vi "LeakageVSTemp-Time_Keithley6517A.vi"() -> ()   [LabVIEW 2010]
uses:
  <vilib>/Instr/_visa.llb/VISA Configure Serial Port (Instr).vi
  <vilib>/Utility/file.llb/Write To Spreadsheet File (DBL).vi
  Instance          14 32Saved   K vs Temp - freq (4284A) .vi
  Instance          10 32Saved   K vs Temp - freq (4284A) .vi
  Instance          25 32Saved   K vs Temp - freq (4284A) .vi
  Instance          24 32Saved   K vs Temp - freq (4284A) .vi
  Instance          26 32Saved   K vs Temp - freq (4284A) .vi
panel:
  in  "Time":dbl[](array[numeric])
  out "?":string="Current"
  in  "control":sgl[](array[numeric]) format="%.2f"
  out "Test Data":sgl[][](array[numeric])=[[1.0, 2.2355776e-13]] format="%.6p"
  out "error out":T1
  in  "error in":T1
  in  "Interval(secs)":sgl=1.0 min=0 max=9999.9 step=0.1 format="%.1f"
  in  "Number of Points":sgl=1.0 min=0 max=9999.9 step=0.1 format="%.1f"
  in  "Bias Voltage":sgl=1.0 min=-1000 max=1000 step=0.1 format="%.1f"
  in  "Current (nA)":dbl[](array[numeric])
  in  "Current (nA)":dbl[](array[numeric])
  in  "Temperature":dbl[](array[numeric])
  in  "Start":bool
  out "Thickness":dbl
  out "Area":dbl
  in  "stop":bool
  out "Temp25Hz":dbl format="%#_3g"
  out "Current (nA) vs. Time":cluster{"Y":dbl[], "Y":dbl[]}[](graph)
  out "Current (nA) vs. Temperature":cluster{"Y":dbl[], "Y":dbl[]}[](graph)
  in  "Comment (Sample's Name, compositions, whatever you want,..)":string
  in  "Thickness (mm)":dbl
  in  "Diameter (mm)":dbl
  in  "Path & File Name (*.txt)":path
  # "Temperature (C)"
  # "Sample Details"
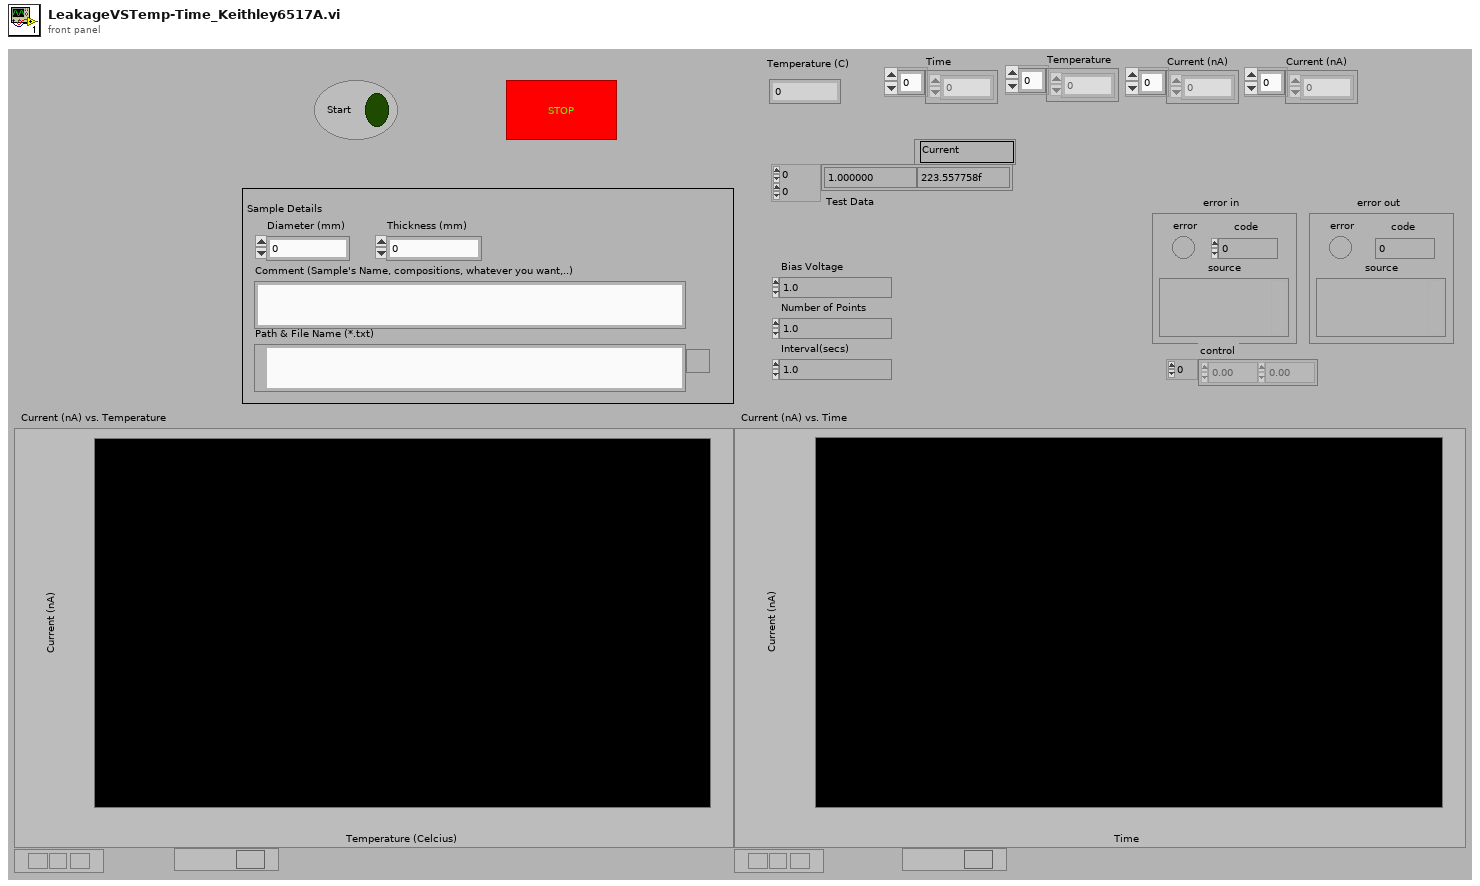
[diagram p1: front panel]
types:
  T1 = cluster{"error":bool, "code":i32, "source":string}
  T2 = cluster{"second":i32, "minute":i32, "hour":i32, "day of month":i32, "month":i32, "year":i32, "day of week":i32, "day of year":i32, "is DST":i32}
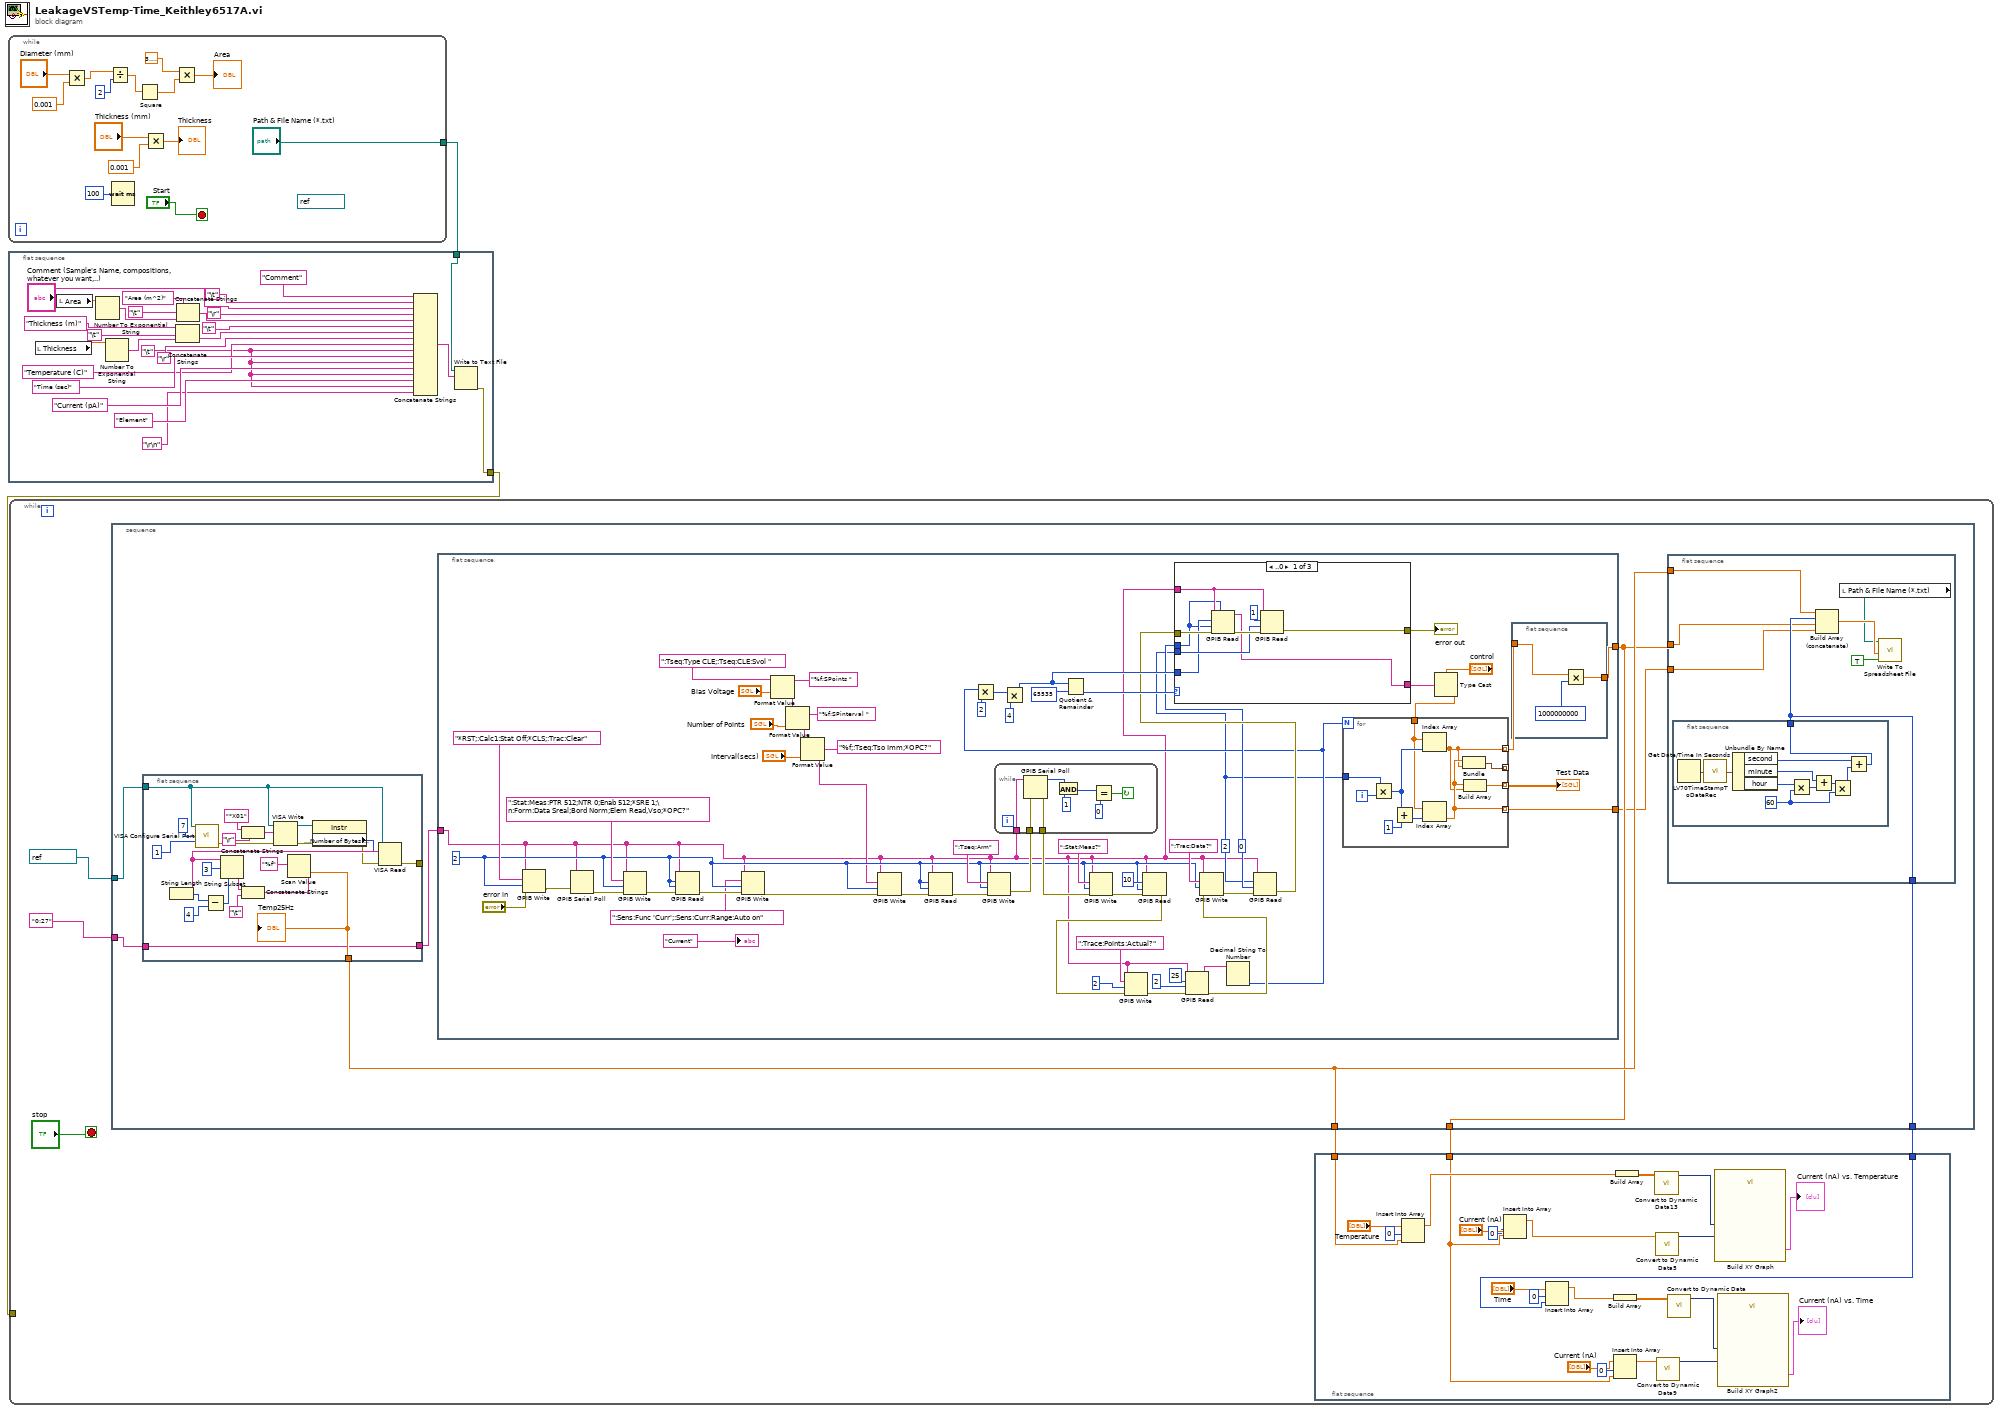
[diagram p0: block diagram]
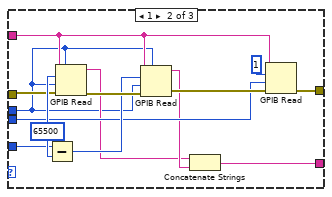
[diagram p2: hidden frame]
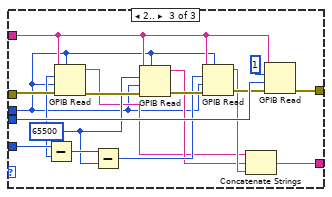
[diagram p3: hidden frame]
diagram:
  n1 = while {
    tunnel: ["Path & File Name (*.txt)"] -> w2
    stop <- "Start" stop-if-true
    (unwired) refnum<visa-resource-name> "COM1" ("VISA Omega (Serial - COM1)")
    n2 = Multiply(x="Diameter (mm)", y=0.001) -> (x*y=w11:dbl)
    n3 = Divide(x=w11, y=2) -> (x/y=w6:dbl)
    n4 = Wait (ms)(milliseconds to wait=u32 100) -> ()  [unwired: 1 out]
    n5 = Square(x=w6) -> (x^2=w7:dbl)
    n6 = Multiply(x="Thickness (mm)", y=0.001) -> (x*y=→"Thickness":dbl)
    n7 = Multiply(x=3.141592653589793, y=w7) -> (x*y=→"Area":dbl)
  }
  n8 = flat-sequence {
    tunnel: w2 -> [w36]
    tunnel: [w34] -> w1
    frame #0 {
      w18 = "\t"
      n9 = local read "Thickness"() -> (w40:dbl)
      n10 = local read "Area"() -> (w41:dbl)
      n11 = Number To Exponential String(number=w41) -> (E-format string=w33:string)  [unwired: 3 in]
      n12 = Number To Exponential String(number=w40) -> (E-format string=w31:string)  [unwired: 3 in]
      n13 = Concatenate Strings("Thickness (m)" ("string"), "\t", w31) -> (w29:string)
      n14 = Concatenate Strings("Area (m^2)" ("string"), "\t", w33) -> (w37:string)
      n15 = Concatenate Strings("Comment" ("string"), "\t", "Comment (Sample's Name, compositions, whatever you want,..)", "\r", w37, "\t", w29, "\r", "Temperature (C)" ("string"), w18, "Time (sec)" ("string"), w18, "Current (pA)" ("string"), w18, "Element" ("string"), w18, "\r\n") -> (w35:string)
      n16 = Write to Text File(file (use dialog)=w36, text=w35) -> (error out=w34:errorcluster)  [unwired: 2 in, 2 out]
    }
  }
  n17 = while {
    tunnel: w1 -> [_]
    stop <- "stop" stop-if-true
    n18 = stacked-sequence {
      tunnel: refnum<visa-resource-name> "COM1" ("VISA Omega (Serial - COM1)") -> [w77]
      tunnel: "0:27" -> [w76]
      tunnel: [w74] -> w44
      tunnel: [w73] -> w43
      tunnel: [w71] -> w42
      frame #0 {
        n19 = flat-sequence {
          tunnel: w77 -> [w217]
          tunnel: [w216] -> _
          tunnel: [w215] -> w74
          tunnel: w76 -> [w214]
          tunnel: [w214] -> w75
          frame #0 {
            n20 = call-poly "VISA Configure Serial Port"("VISA resource name"=w217, "data bits (8)"=7, "parity (0:none)"=1) -> ("error out"=w222:errorcluster)  [unwired: 11 in, 1 out]
            n21 = Concatenate Strings("*X01", "\r") -> (w225:string)
            n22 = VISA Write(VISA resource name=w217, write buffer=w225, error in (no error)=w222) -> (VISA resource name out=w236:refnum<visa-resource-name>, error out=w226:errorcluster)  [unwired: 1 out]
            n23 = property class="Instr"(reference=w236, error in=w226) -> (error out=w227:errorcluster, "Serial Settings:Number of Bytes at Serial Port"=w228:u32)  [unwired: 1 out]
            n24 = VISA Read(VISA resource name=w217, byte count=w228, error in (no error)=w227) -> (read buffer=w229:string, error out=w216:errorcluster)  [unwired: 2 out]
            n25 = String Length(string=w229) -> (length=w231:i32)
            n26 = Subtract(x=w231, y=4) -> (x-y=w233:i32)
            n27 = String Subset(string=w229, offset (0)=3, length (rest)=w233) -> (substring=w234:string)
            n28 = Concatenate Strings(w234, "\t") -> (w218:string)
            n29 = Scan Value(string=w218, format string="%f") -> (value=w215:dbl)  [unwired: 1 in, 1 out]
            "Temp25Hz" <- w215
          }
        }
        n30 = flat-sequence {
          tunnel: w75 -> [w98]
          tunnel: [w97] -> w72
          tunnel: [w95] -> w73
          frame #0 {
            w124 = 0
            w109 = 2
            w102 = 2
            n31 = GPIB Write(0:w98, 1:"*RST;:Calc1:Stat Off;*CLS;:Trac:Clear", 2:w102, 3:"error in") -> (6:w150:errorcluster)  [unwired: 1 in, 1 out]
            n32 = GPIB Serial Poll(0:w98, 1:w150) -> (4:w149:errorcluster)  [unwired: 2 out]
            n33 = GPIB Write(0:w98, 1:":Stat:Meas:PTR 512;NTR 0;Enab 512;*SRE 1;\n:Form:Data Sreal;Bord Norm;Elem Read,Vso;*OPC?", 2:w102, 3:w149) -> (6:w147:errorcluster)  [unwired: 1 in, 1 out]
            n34 = GPIB Read(0:w98, 1:w102, 2:w102, 3:w147) -> (7:w103:errorcluster)  [unwired: 1 in, 2 out]
            n35 = GPIB Write(0:w98, 1:":Sens:Func 'Curr';:Sens:Curr:Range:Auto on", 2:w102, 3:w103) -> (6:w104:errorcluster)  [unwired: 1 in, 1 out]
            n36 = Format Value(string ("")=":Tseq:Type CLE;:Tseq:CLE:Svol ", format string="%f;SPoints ", value (0)="Bias Voltage") -> (output string=w144:string)
            n37 = Format Value(string ("")=w144, format string="%f;SPinterval ", value (0)="Number of Points") -> (output string=w142:string)
            n38 = Format Value(string ("")=w142, format string="%f;:Tseq:Tso Imm;*OPC?", value (0)="Interval(secs)") -> (output string=w99:string)
            n39 = GPIB Write(0:w98, 1:w99, 2:w102, 3:w104) -> (6:w140:errorcluster)  [unwired: 1 in, 1 out]
            n40 = GPIB Read(0:w98, 1:w102, 2:w102, 3:w140) -> (7:w139:errorcluster)  [unwired: 1 in, 2 out]
            n41 = GPIB Write(0:w98, 1:":Tseq:Arm", 2:w102, 3:w139) -> (6:w132:errorcluster)  [unwired: 1 in, 1 out]
            n42 = while {
              tunnel: w132 -> [w209]
              tunnel: [w208] -> w131
              tunnel: w98 -> [w207]
              stop <- w212 continue-if-true
              n43 = GPIB Serial Poll(0:w207, 1:w209) -> (2:w211:i16, 4:w208:errorcluster)  [unwired: 1 out]
              n44 = And(x=w211, y=1) -> (x .and. y?=w206:i32)
              n45 = Equal?(x=w206, y=0) -> (x = y?=w212:bool)
            }
            n46 = GPIB Write(0:w98, 1:":Stat:Meas?", 2:w102, 3:w131) -> (6:w136:errorcluster)  [unwired: 1 in, 1 out]
            n47 = GPIB Read(0:w98, 1:10, 2:w102, 3:w136) -> (7:w117:errorcluster)  [unwired: 1 in, 2 out]
            n48 = GPIB Write(0:w98, 1:":Trace:Points:Actual?", 2:2, 3:w117) -> (6:w120:errorcluster)  [unwired: 1 in, 1 out]
            n49 = GPIB Read(0:w98, 1:25, 2:2, 3:w120) -> (5:w115:string, 7:w116:errorcluster)  [unwired: 1 in, 1 out]
            n50 = GPIB Write(0:w98, 1:":Trac:Data?", 2:w102, 3:w116) -> (6:w133:errorcluster)  [unwired: 1 in, 1 out]
            n51 = Decimal String To Number(string=w115) -> (number=w110:i32)  [unwired: 2 in, 1 out]
            n52 = Multiply(x=w110, y=2) -> (x*y=w111:i32)
            n53 = Multiply(x=w111, y=4) -> (x*y=w127:i32)
            n54 = Quotient & Remainder(x=w127, y=65535) -> (floor(x/y)=w128:i32)  [unwired: 1 out]
            n55 = GPIB Read(0:w98, 1:w109, 2:w124, 3:w133) -> (7:w125:errorcluster)  [unwired: 1 in, 2 out]
            n56 = case shown="..0" w128 {
              tunnel: w125 -> [w172 w180 w202]
              tunnel: w109 -> [w171 w182 w204]
              tunnel: [w170 w179 w194] -> w108
              tunnel: [w169 w183 w203] -> w123
              tunnel: w127 -> [w168 w181 w200]
              tunnel: w98 -> [w167 w176 w190]
              tunnel: w124 -> [w166 w175 w189]
              frame ..0 {
                n57 = GPIB Read(0:w167, 1:w168, 2:w166, 3:w172, 4:w166) -> (5:w170:string, 7:w173:errorcluster)  [unwired: 1 out]
                n58 = GPIB Read(0:w167, 1:1, 2:w171, 3:w173) -> (7:w169:errorcluster)  [unwired: 1 in, 2 out]
              }
              frame 1 {
                w185 = 65500
                n59 = Subtract(x=w181, y=w185) -> (x-y=w184:i32)
                n60 = GPIB Read(0:w176, 1:w185, 2:w175, 3:w180, 4:w175) -> (5:w177:string, 7:w187:errorcluster)  [unwired: 1 out]
                n61 = GPIB Read(0:w176, 1:w184, 2:w175, 3:w187, 4:w175) -> (5:w178:string, 7:w186:errorcluster)  [unwired: 1 out]
                n62 = Concatenate Strings(w177, w178) -> (w179:string)
                n63 = GPIB Read(0:w176, 1:1, 2:w182, 3:w186) -> (7:w183:errorcluster)  [unwired: 1 in, 2 out]
              }
              frame 2.. {
                w196 = 65500
                n64 = Subtract(x=w200, y=w196) -> (x-y=w197:i32)
                n65 = GPIB Read(0:w190, 1:w196, 2:w189, 3:w202, 4:w189) -> (5:w191:string, 7:w201:errorcluster)  [unwired: 1 out]
                n66 = Subtract(x=w197, y=w196) -> (x-y=w195:i32)
                n67 = GPIB Read(0:w190, 1:w196, 2:w189, 3:w201, 4:w189) -> (5:w192:string, 7:w198:errorcluster)  [unwired: 1 out]
                n68 = GPIB Read(0:w190, 1:w195, 2:w189, 3:w198, 4:w189) -> (5:w193:string, 7:w199:errorcluster)  [unwired: 1 out]
                n69 = Concatenate Strings(w191, w192, w193) -> (w194:string)
                n70 = GPIB Read(0:w190, 1:1, 2:w204, 3:w199) -> (7:w203:errorcluster)  [unwired: 1 in, 2 out]
              }
            }
            "error out" <- w123
            n71 = Type Cast(type="control", x=w108) -> (*(type *) &x=w107:sgl[])
            n72 = for {
              N: w110 -> [_]
              tunnel: w109 -> [w164]
              tunnel: w107 -> [w160]
              tunnel: [w159] -> w105 mode=indexing
              tunnel: [w158] -> _ mode=indexing
              tunnel: [w157] -> w97 mode=indexing
              tunnel: [w156] -> w96 mode=indexing
              i -> [w163]
              n73 = Multiply(x=w164, y=w163) -> (x*y=w162:i32)
              n74 = Add(x=w162, y=1) -> (x+y=w161:i32)
              n75 = Index Array(array=w160, index=w162) -> (element=w156:sgl)
              n76 = Index Array(array=w160, index=w161) -> (element=w157:sgl)
              n77 = Bundle("Current"=w157, "Current"=w156) -> (w158:cluster{"Current":sgl, "Current":sgl})  [unwired: 1 in]
              n78 = Build Array(w157, w156) -> (w159:sgl[])
            }
            "Test Data" <- w105
            n79 = flat-sequence {
              tunnel: w96 -> [w155]
              tunnel: [w154] -> w95
              frame #0 {
                n80 = Multiply(x=w155, y=1000000000) -> (x*y=w154:sgl[])
              }
            }
            "?" <- "Current"
          }
        }
        n81 = flat-sequence {
          tunnel: w74 -> [w81]
          tunnel: w72 -> [w78]
          tunnel: w73 -> [w79]
          tunnel: [w80] -> w71
          frame #0 {
            n82 = flat-sequence {
              tunnel: [w85] -> w80
              frame #0 {
                w87 = 60
                n83 = Get Date/Time In Seconds() -> (seconds since 1Jan1904=w86:timestamp)
                n84 = call <vilib>:"LV70TimeStampToDateRec.vi"("time stamp"=w86) -> ("date time rec"=w94:T2)
                n85 = Unbundle By Name(w94) -> ("second"=w88:i32, "minute"=w91:i32, "hour"=w93:i32)
                n86 = Multiply(x=w93, y=w87) -> (x*y=w92:i32)
                n87 = Add(x=w91, y=w92) -> (x+y=w90:i32)
                n88 = Multiply(x=w90, y=w87) -> (x*y=w89:i32)
                n89 = Add(x=w88, y=w89) -> (x+y=w85:i32)
              }
            }
            n90 = Build Array (concatenate)(w81, w80, w79, w78) -> (w84:dbl[])
            n91 = local read "Path & File Name (*.txt)"() -> (w82:path)
            n92 = call-poly <vilib>:"Write To Spreadsheet File.vi"("append to file? (new file:F)"=TRUE, "1D data"=w84, "file path (dialog if empty)"=w82) -> ()  [unwired: 5 in, 1 out]
          }
        }
      }
    }
    n93 = flat-sequence {
      tunnel: w44 -> [w61]
      tunnel: w43 -> [w54]
      tunnel: w42 -> [w51]
      frame #0 {
        n94 = Insert Into Array(array="Temperature", index=0, new element=w61) -> (w55:dbl[])
        n95 = Insert Into Array(array="Current (nA)", index=0, new element=w54) -> (w60:dbl[])
        n96 = Insert Into Array(array="Time", index=0, new element=w51) -> (w50:dbl[])
        n97 = Insert Into Array(array="Current (nA)", index=0, new element=w54) -> (w67:dbl[])
        n98 = Build Array(w50) -> (w49:dbl[][])
        n99 = Build Array(w55) -> (w59:dbl[][])
        n100 = call "Convert to Dynamic Data13"("2D Array"=w59) -> ("Dynamic Data Type"=w56:dynamicdata)  [unwired: 3 in]
        n101 = call "Convert to Dynamic Data5"("Array"=w60) -> ("Dynamic Data Type"=w57:dynamicdata)  [unwired: 3 in]
        n102 = call "Convert to Dynamic Data9"("Array"=w67) -> ("Dynamic Data Type"=w58:dynamicdata)  [unwired: 3 in]
        n103 = call "Convert to Dynamic Data"("2D Array"=w49) -> ("Dynamic Data Type"=w48:dynamicdata)  [unwired: 3 in]
        n104 = call "Build XY Graph"("Y Input"=w57, "X Input"=w56) -> ("XY Graph"=→"Current (nA) vs. Temperature":cluster{"Y":dbl[], "Y":dbl[]}[])  [unwired: 8 in, 1 out]
        n105 = call "Build XY Graph2"("Y Input"=w58, "X Input"=w48) -> ("XY Graph"=→"Current (nA) vs. Time":cluster{"Y":dbl[], "Y":dbl[]}[])  [unwired: 8 in, 1 out]
      }
    }
  }
